vi "WriteSpeedProfile.vi"(8 "error in (no error)":errorcluster, 11 "TDMS File":path) -> (0 "error out":errorcluster, 3 "TDMS File Out":path)   [LabVIEW 2017]
uses:
  <vilib>/addons/Sound and Vibration/Order Analysis/Tach Process/SVPO Analog Tacho Process (1 Ch DBL Array).vi
  <vilib>/addons/Sound and Vibration/Order Analysis/Tach Process/SVPO Analog Tacho Process (1 Ch DBL Array) with IC.vi
  <vilib>/addons/Sound and Vibration/Order Analysis/Tach Process/SubVIs/oa_Convert Pulse Positions to Speed (No State).vi
  <vilib>/addons/Sound and Vibration/Order Analysis/Tach Process/SubVIs/sv_Edge Detection (1 Tach) with IC.vi
  <vilib>/addons/Sound and Vibration/Order Analysis/Tach Process/SubVIs/oa_Analog Tacho Hysteresis(1 Channel) with IC.vi
  <vilib>/addons/_NISVFA/_Shared subVIs/Common/SV Buffer Array (No State) (DBL).vi
  <vilib>/addons/Sound and Vibration/Order Analysis/Tach Process/SubVIs/OAT Cross Point Detection.vi
  <vilib>/addons/_NISVFA/_Shared subVIs/Common/svc_Get Array Subset (Index).vi
  <vilib>/Analysis/8numeric.llb/Threshold Detector.vi
  <vilib>/addons/_NISVFA/_Shared subVIs/Common/svc_Coerce Index and Length.vi
  <vilib>/addons/_NISVFA/_Shared subVIs/Common/svc_Conditional Merge Error.vi
  <vilib>/addons/Sound and Vibration/Order Analysis/Tach Process/SoundVib_TachProcess.lvlib
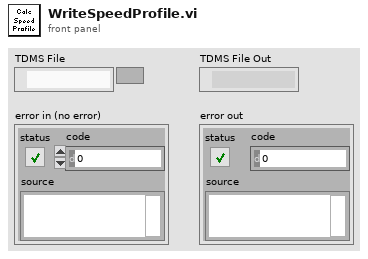
[diagram p1: front panel]
types:
  T1 = typedef "OAT Position Info.ctl" = cluster{"positions [s]":dbl[], "samples/rev":dbl}
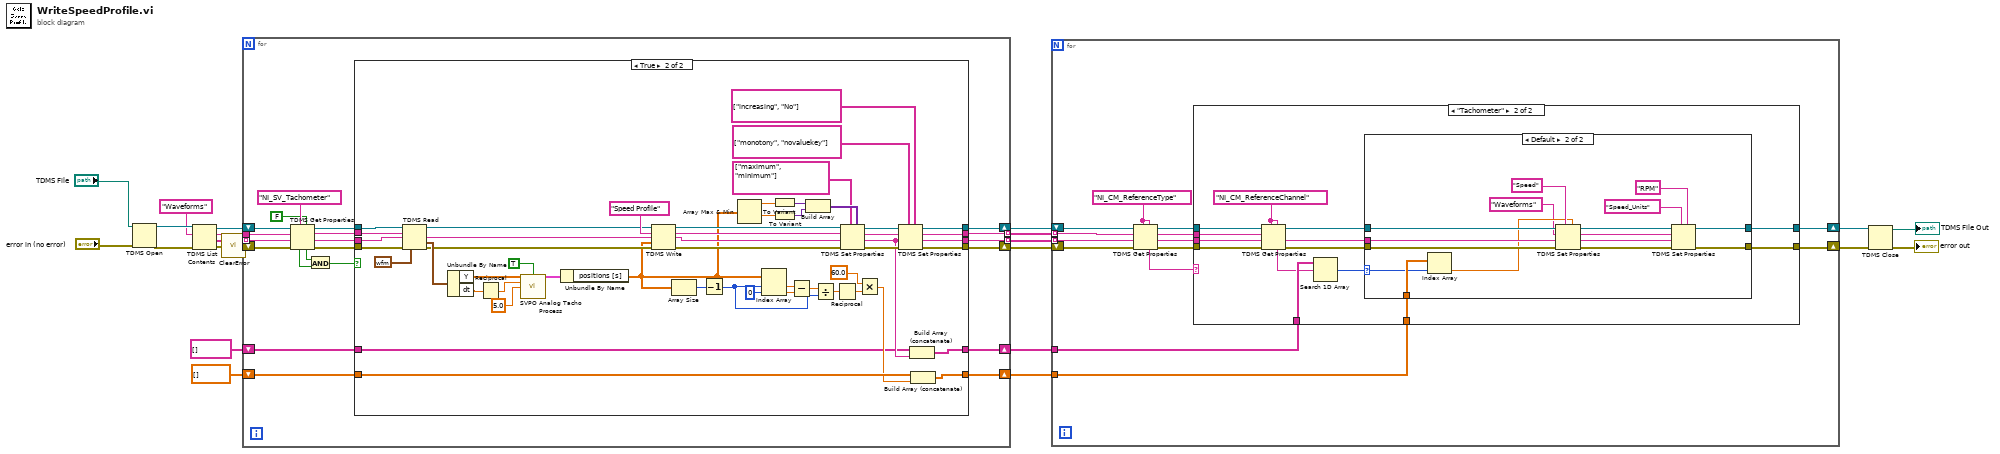
[diagram p0: block diagram]
diagram:
  n1 = TDMS Open(8:"error in (no error)", 11:"TDMS File") -> (0:w21:errorcluster, 3:w22:refnum<k34>)  [unwired: 5 in]
  n2 = TDMS List Contents(4:w21, 6:"Waveforms" ("group name"), 7:w22) -> (0:w1:errorcluster, 1:w15:string[], 2:w16:string, 3:w17:refnum<k34>)
  n3 = call <vilib>:"ClearError.vi"("error in (no error)"=w1) -> ("error out"=w14:errorcluster)
  n4 = for {
    tunnel: w16 -> [w41]
    tunnel: w15 -> [w40] mode=indexing
    shift-right: [w30] -> w5
    shift-left: dbl[] [] -> [w29]
    shift-right: [w27] -> w6
    shift-left: string[] [] -> [w28]
    shift-right: [w26] -> w9
    shift-left: w14 -> [w43]
    tunnel: [w25] -> w8 mode=indexing
    tunnel: [w24] -> w7 mode=indexing
    shift-right: [w23] -> w2
    shift-left: w17 -> [w42]
    n5 = TDMS Get Properties(5:FALSE ("found"), 7:"NI_SV_Tachometer" ("property name"), 8:w43, 9:w40, 10:w41, 11:w42) -> (0:w34:errorcluster, 1:w31:string, 2:w32:string, 3:w33:refnum<k34>, 4:w37:bool, 6:w36:bool)
    n6 = And(x=w37, y=w36) -> (x .and. y?=w35:bool)
    n7 = case shown="True" w35 {
      tunnel: w34 -> [w46 w100]
      tunnel: w33 -> [w47 w99]
      tunnel: w32 -> [w44 w98]
      tunnel: w31 -> [w45 w97]
      tunnel: [w49 w57] -> w30
      tunnel: w29 -> [w49 w59]
      tunnel: w28 -> [w48 w55]
      tunnel: [w48 w54] -> w27
      tunnel: [w46 w53] -> w26
      tunnel: [w47 w52] -> w23
      tunnel: [w45 w50] -> w25
      tunnel: [w44 w51] -> w24
      frame False {
      }
      frame True {
        n8 = TDMS Read(0:w99, 5:w98, 7:w97, 11:w100, 12:waveform(sgl) {"t0"=timestamp(0 s since 1904-01-01), "dt"=1.0, "Y"=[]} ("data type")) -> (4:w85:refnum<k34>, 8:w87:string, 10:w95:waveform(sgl), 15:w88:errorcluster)  [unwired: 3 in, 2 out]
        n9 = Unbundle By Name(w95) -> ("Y"=w94:sgl[], "dt"=w93:dbl)
        n10 = Reciprocal(x=w93) -> (1/x=w92:dbl)
        n11 = call-poly <vilib>:"SVPO Analog Tacho Process.vi"("analog tacho signal"=w94, "reset? (F)"=TRUE, "sampling rate [Hz]"=w92, "threshold"=5.0) -> ("speed position info"=w89:T1)  [unwired: 10 in, 1 out]
        n12 = Unbundle By Name(w89) -> ("positions [s]"=w61:dbl[])
        n13 = TDMS Write(0:w85, 5:"Speed Profile" ("group name in (Untitled)"), 7:w87, 9:w61, 11:w88) -> (4:w70:refnum<k34>, 6:w71:string, 8:w72:string, 15:w73:errorcluster)  [unwired: 1 in]
        n14 = Array Size(array=w61) -> (size(s)=w65:i32)
        n15 = Decrement(x=w65) -> (x-1=w64:i32)
        n16 = Array Max & Min(array=w61) -> (max value=w75:dbl, min value=w76:dbl)  [unwired: 2 out]
        n17 = Index Array(array=w61, index #1=w64, index #2=0 ("index")) -> (element #1=w60:dbl, element #2=w62:dbl)
        n18 = To Variant(anything=w75) -> (Variant=w77:variant)
        n19 = To Variant(anything=w76) -> (Variant=w78:variant)
        n20 = Subtract(x=w60, y=w62) -> (x-y=w68:dbl)
        n21 = Build Array(w77, w78) -> (w79:variant[])
        n22 = Divide(x=w68, y=w64) -> (x/y=w67:dbl)
        n23 = Reciprocal(x=w67) -> (1/x=w63:dbl)
        n24 = TDMS Set Properties(5:w79, 7:string[] ["maximum", "minimum"] ("property names"), 8:w73, 9:w72, 10:w71, 11:w70) -> (0:w80:errorcluster, 1:w56:string, 2:w81:string, 3:w82:refnum<k34>)
        n25 = Multiply(x=60.0, y=w63) -> (x*y=w58:dbl)
        n26 = TDMS Set Properties(5:string[] ["increasing", "No"] ("property names"), 7:string[] ["monotony", "novaluekey"] ("property names"), 8:w80, 9:w56, 10:w81, 11:w82) -> (0:w53:errorcluster, 1:w50:string, 2:w51:string, 3:w52:refnum<k34>)
        n27 = Build Array (concatenate)(w55, w56) -> (w54:string[])
        n28 = Build Array (concatenate)(w59, w58) -> (w57:dbl[])
      }
    }
  }
  n29 = for {
    shift-right: [w103] -> w4
    shift-left: w9 -> [w108]
    tunnel: w8 -> [w109] mode=indexing
    tunnel: w7 -> [w107] mode=indexing
    tunnel: w6 -> [w105]
    tunnel: w5 -> [w104]
    shift-right: [w102] -> w3
    shift-left: w2 -> [w106]
    w101 = "NI_CM_ReferenceType" ("property name")
    n30 = TDMS Get Properties(5:w101, 7:w101, 8:w108, 9:w109, 10:w107, 11:w106) -> (0:w111:errorcluster, 1:w114:string, 2:w113:string, 3:w112:refnum<k34>, 4:w110:string)  [unwired: 1 out]
    n31 = case shown="\"Tachometer\"" w110 {
      tunnel: w111 -> [w115 w129]
      tunnel: w112 -> [w116 w130]
      tunnel: w113 -> [_ w128]
      tunnel: w114 -> [_ w127]
      tunnel: w105 -> [_ w126]
      tunnel: w104 -> [_ w124]
      tunnel: [w115 w119] -> w103
      tunnel: [w116 w118] -> w102
      frame Default {
      }
      frame "Tachometer" {
        w117 = "NI_CM_ReferenceChannel" ("property name")
        n32 = TDMS Get Properties(5:w117, 7:w117, 8:w129, 9:w127, 10:w128, 11:w130) -> (0:w121:errorcluster, 1:w120:string, 3:w122:refnum<k34>, 4:w125:string)  [unwired: 2 out]
        n33 = Search 1D Array(1D array=w126, element=w125) -> (index of element=w123:i32)  [unwired: 1 in]
        n34 = case shown="Default" w123 {
          selector: w123 -> [_ w147]
          tunnel: w124 -> [_ w148]
          tunnel: w122 -> [w132 w143]
          tunnel: w121 -> [w131 w146]
          tunnel: w120 -> [_ w145]
          tunnel: [w131 w136] -> w119
          tunnel: [w132 w133] -> w118
          frame -1 {
          }
          frame Default {
            n35 = Index Array(array=w148, index=w147) -> (element=w142:dbl)
            n36 = TDMS Set Properties(5:w142, 7:"Speed" ("property name"), 8:w146, 9:w145, 10:"Waveforms" ("group name"), 11:w143) -> (0:w137:errorcluster, 1:w138:string, 2:w139:string, 3:w140:refnum<k34>)
            n37 = TDMS Set Properties(5:"RPM" ("property name"), 7:"Speed_Units" ("property name"), 8:w137, 9:w138, 10:w139, 11:w140) -> (0:w136:errorcluster, 3:w133:refnum<k34>)  [unwired: 2 out]
          }
        }
      }
    }
  }
  n38 = TDMS Close(8:w4, 11:w3) -> (0:→"error out":errorcluster, 3:→"TDMS File Out":path)
